vi "Move XYZ.vi"(0 "PID Gains In":T2={"X PID"={"proportional gain (Kc)"=0.03, "integral time (Ti, min)"=0.0, "derivative time (Td, min)"=0.0}, "Y PID"={"proportional gain (Kc)"=0.03, "integral time (Ti, min)"=0.0, "derivative time (Td, min)"=0.0}, "Z PID"={"proportional gain (Kc)"=0.035, "integral time (Ti, min)"=0.0, "derivative time (Td, min)"=0.0}} {"Z PID"."derivative time (Td, min)" format="%.3f"; "Z PID"."integral time (Ti, min)" format="%.3f"; "Z PID"."proportional gain (Kc)" format="%.3f"; "Y PID"."derivative time (Td, min)" format="%.3f"; "Y PID"."integral time (Ti, min)" format="%.3f"; "Y PID"."proportional gain (Kc)" format="%.3f"; "X PID"."derivative time (Td, min)" format="%.3f"; "X PID"."integral time (Ti, min)" format="%.3f"; "X PID"."proportional gain (Kc)" format="%.3f"}, 5 "Y Target":dbl, 6 "X Target":dbl, 10 "Max Time":dbl=90.0, 11 "Gyro Target":dbl=-180.0, 12 "Movement":dbl=3.0, 14 "X Output Range":cluster{"output high":dbl, "output low":dbl}={"output high"=0.8, "output low"=-0.8}, 15 "X Stop Threshold":dbl=5.0, 16 "Y Output Range":cluster{"output high":dbl, "output low":dbl}={"output high"=0.8, "output low"=-0.8}, 17 "Y Stop Threshold":dbl=5.0, 18 "Z Output Range":cluster{"output high":dbl, "output low":dbl}={"output high"=0.8, "output low"=-0.8}, 19 "Z  Stop Threshold":dbl=8.0) -> ()   [LabVIEW 2018]
uses:
  Robot Global Data.vi
  SubSystems/Drive Train/Drive Train Global.vi
  SubSystems/Hatch Panel Intake/Hatch Panel Intake Global.vi
  SubSystems/Lift/Lift Global.vi
  <vilib>/addons/control/pid/pid.llb/PID (DBL).vi
  <vilib>/addons/control/pid/NI_PID_pid.lvlib
panel:
  in  "Camera Tracking":T1={"proportional gain (Kc)"=0.06, "integral time (Ti, min)"=0.0, "derivative time (Td, min)"=0.0}
  in  "Minimum Time":u32=500
  in  "Settle Time":u32=2000
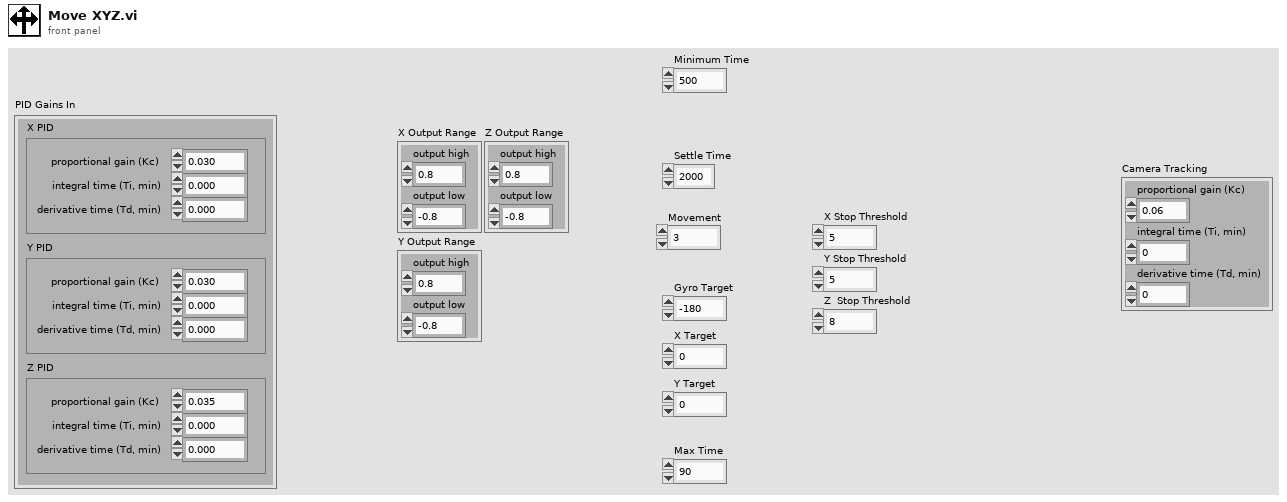
[diagram p1: front panel]
types:
  T1 = cluster{"proportional gain (Kc)":dbl, "integral time (Ti, min)":dbl, "derivative time (Td, min)":dbl}
  T2 = cluster{"X PID":cluster{"proportional gain (Kc)":dbl, "integral time (Ti, min)":dbl, "derivative time (Td, min)":dbl}, "Y PID":cluster{"proportional gain (Kc)":dbl, "integral time (Ti, min)":dbl, "derivative time (Td, min)":dbl}, "Z PID":cluster{"proportional gain (Kc)":dbl, "integral time (Ti, min)":dbl, "derivative time (Td, min)":dbl}}
  T3 = cluster{"Rollover":dbl, "Yaw":dbl, "Cont Yaw":dbl}
  T4 = cluster{"offsetAngle H":dbl, "offsetAngle V":dbl, "area":dbl, "skew":dbl, "validTarget":dbl, "latency":dbl}
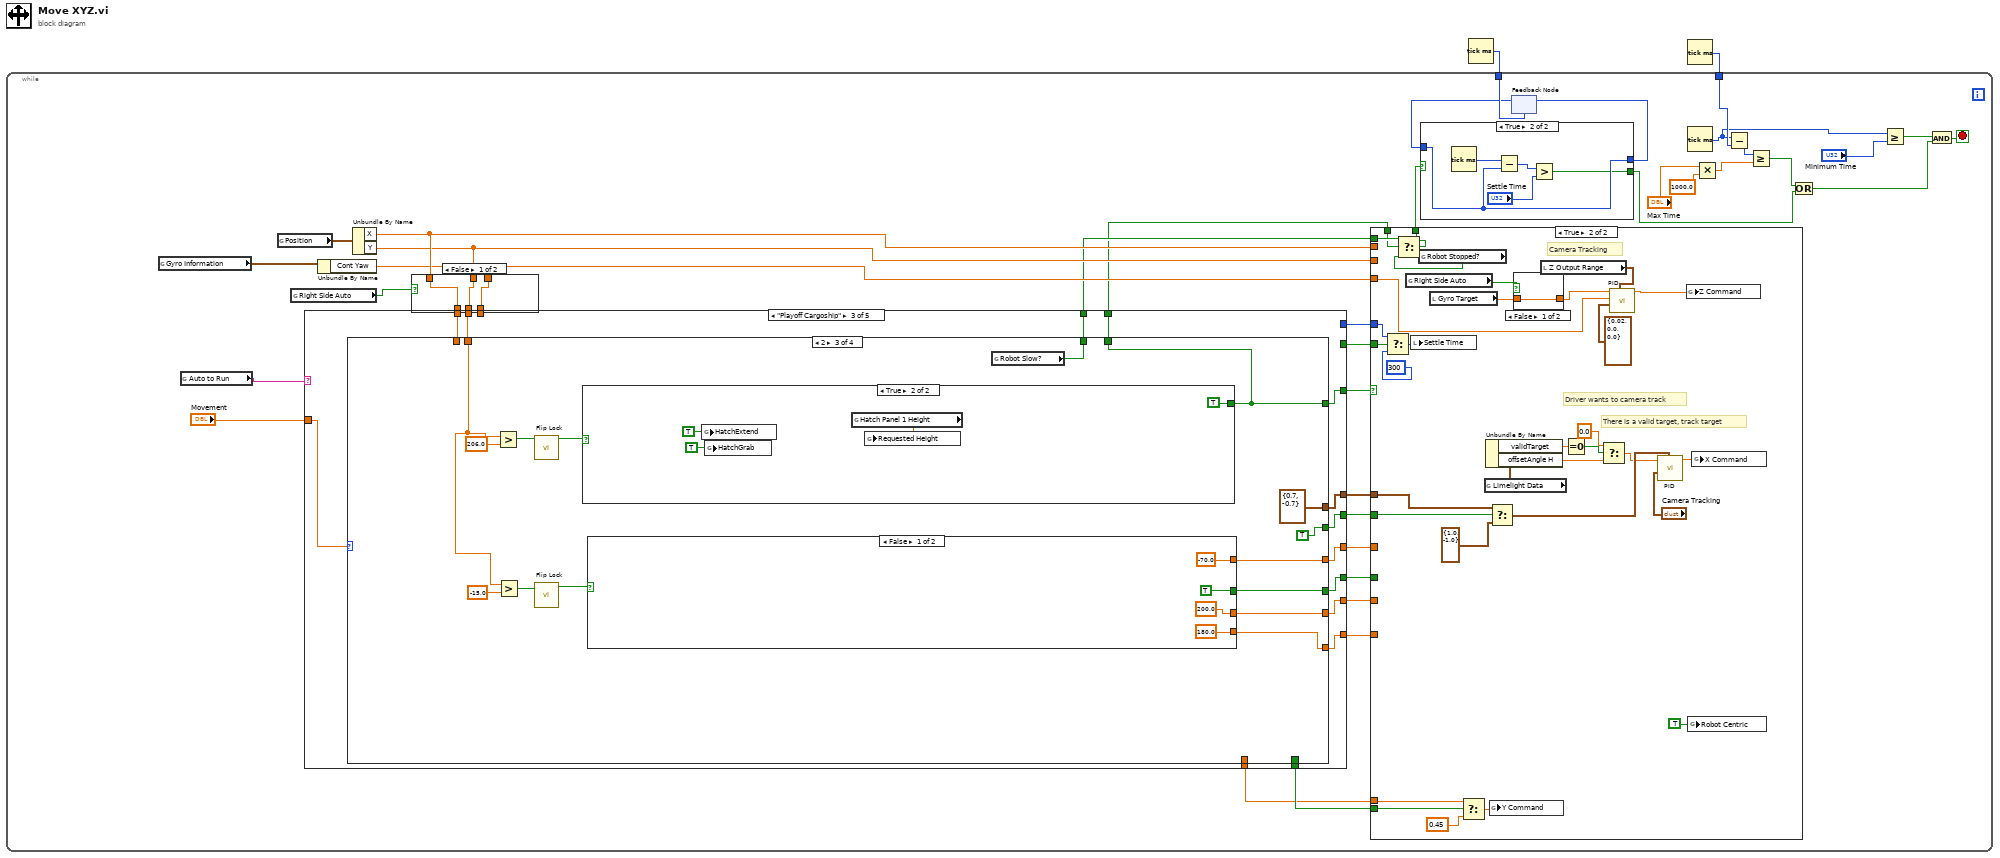
[diagram p0: block diagram]
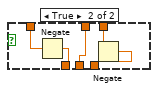
[diagram p2: hidden frame]
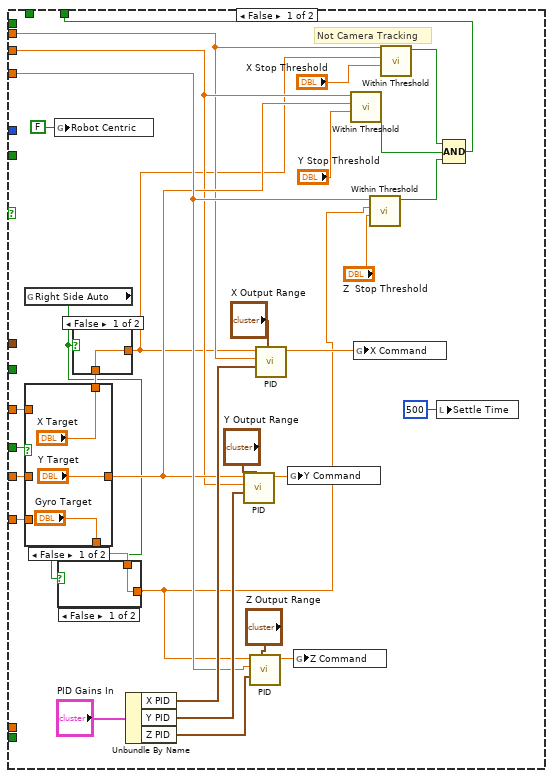
[diagram p3: hidden frame]
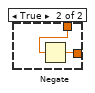
[diagram p4: hidden frame]
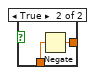
[diagram p5: hidden frame]
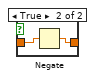
[diagram p7: hidden frame]
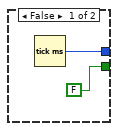
[diagram p8: hidden frame]
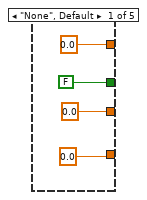
[diagram p9: hidden frame]
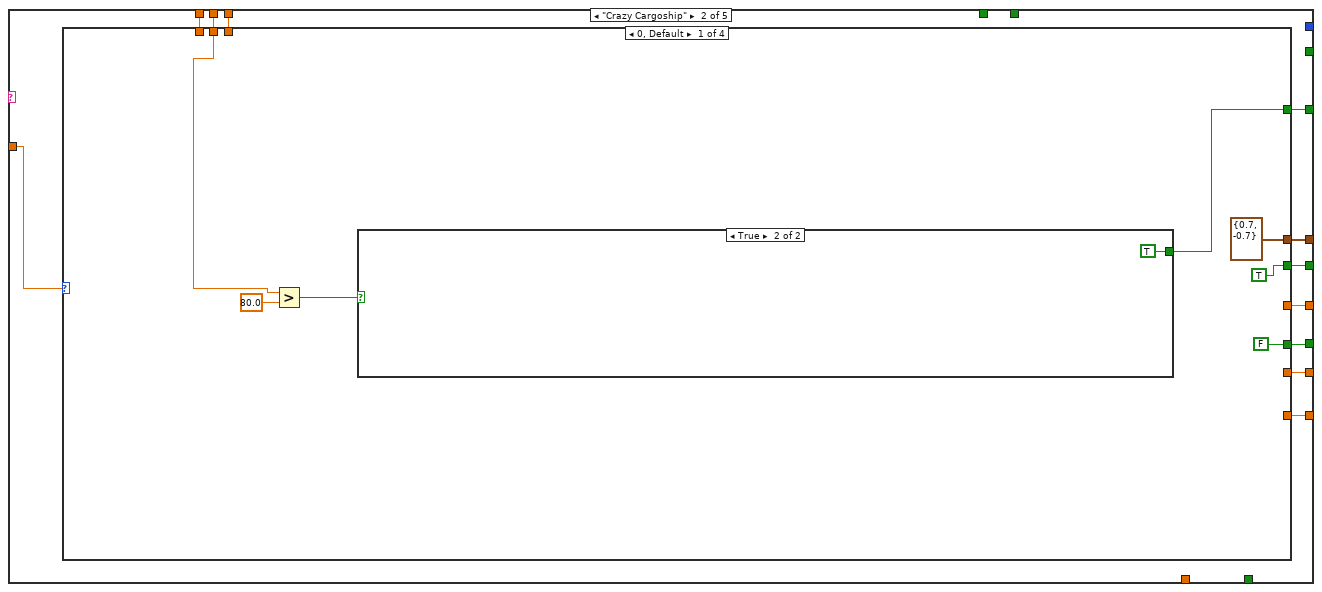
[diagram p10: hidden frame]
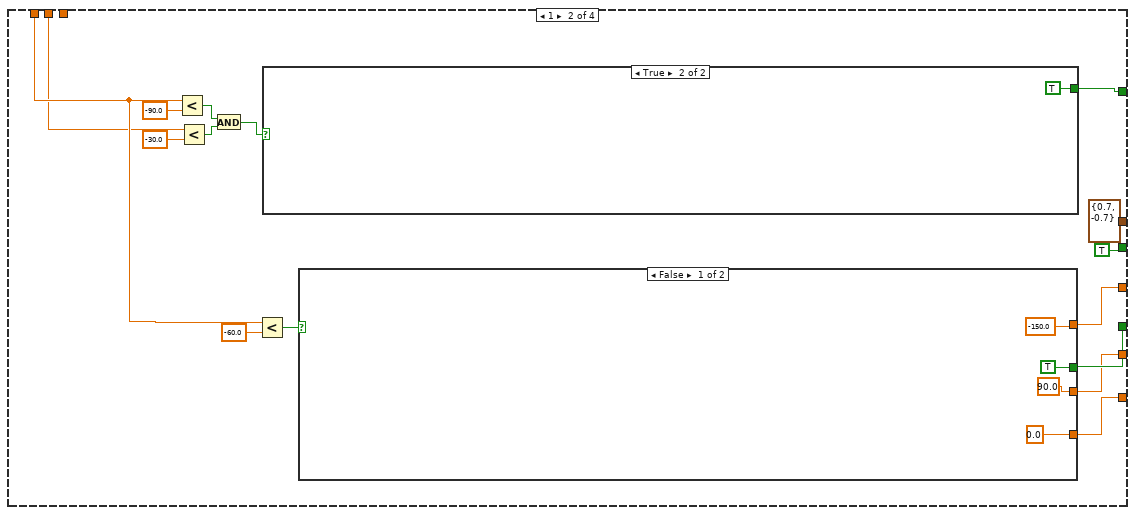
[diagram p12: hidden frame]
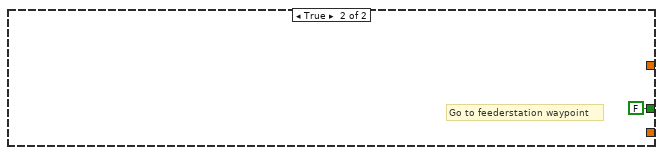
[diagram p13: hidden frame]
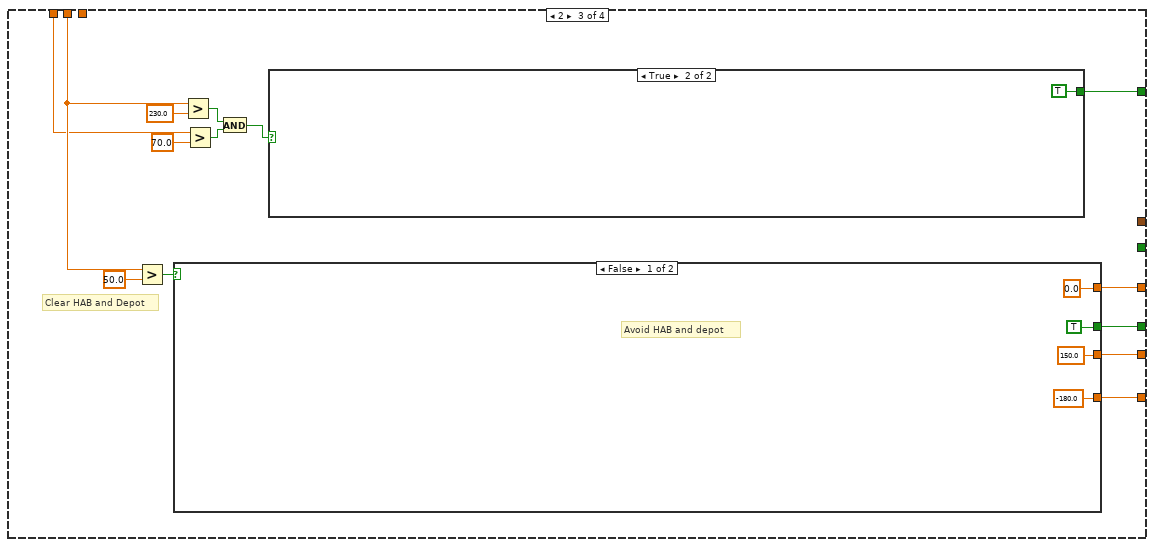
[diagram p15: hidden frame]
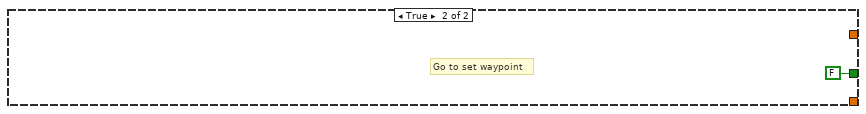
[diagram p17: hidden frame]
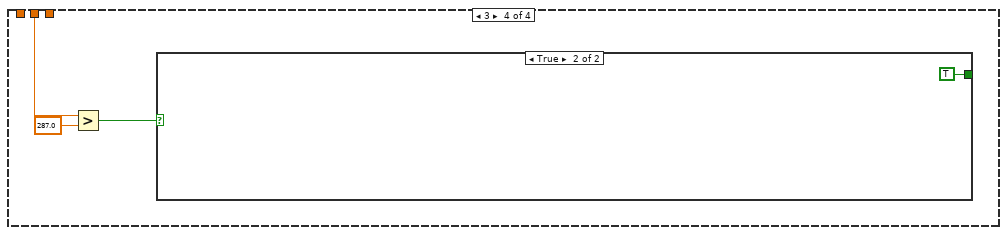
[diagram p18: hidden frame]
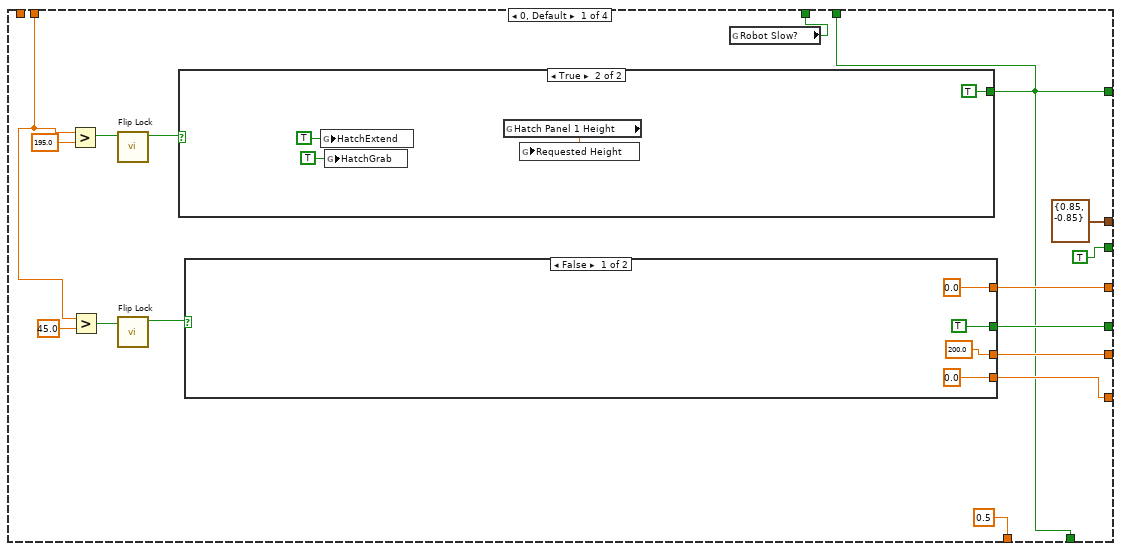
[diagram p20: hidden frame]
diagram:
  n1 = Tick Count (ms)() -> (millisecond timer value=w2:u32)
  n2 = Tick Count (ms)() -> (millisecond timer value=w1:u32)
  n3 = while {
    tunnel: w2 -> [w36]
    tunnel: w1 -> [w24]
    stop <- w23 stop-if-true
    n4 = global read "Drive Train Global.vi" "Gyro Information"() -> (w30:T3)
    n5 = global read "Robot Global Data.vi" "Auto to Run"() -> (w33:string)
    n6 = global read "Drive Train Global.vi" "Position"() -> (w32:cluster{"X":dbl, "Y":dbl})
    n7 = global read "Robot Global Data.vi" "Right Side Auto"() -> (w7:bool)
    n8 = Unbundle By Name(w30) -> ("Cont Yaw"=w9:dbl)
    n9 = Unbundle By Name(w32) -> ("X"=w12:dbl, "Y"=w10:dbl)
    n10 = case shown="False" w7 {
      tunnel: [w45 w50] -> w13
      tunnel: w12 -> [w45 w49]
      tunnel: [w44 w48] -> w11
      tunnel: w10 -> [w44 w48]
      tunnel: w9 -> [w43 w47]
      tunnel: [w43 w46] -> w8
      frame False {
      }
      frame True {
        n11 = Negate(x=w49) -> (-x=w50:dbl)
        n12 = Negate(x=w47) -> (-x=w46:dbl)
      }
    }
    n13 = case shown="\"Playoff Cargoship\"" w33 {
      tunnel: [0.0 w146 w213 w308 w403] -> w42
      tunnel: [0.0 w145 w211 w307 w402] -> w41
      tunnel: [0.0 w144 w210 w306 w401] -> w40
      tunnel: w11 -> [_ w150 w218 w311 w406]
      tunnel: [FALSE w149 w212 w309 w404] -> w39
      tunnel: w13 -> [_ w147 w219 w310 w405]
      tunnel: "Movement" -> [_ w151 w217 w312 w407]
      tunnel: w8 -> [_ w148 _ _ w399]
      tunnel: [_ w143 w215 w305 w400] -> w18
      tunnel: [_ w141 w216 w303 _] -> w17
      tunnel: [_ w142 w214 w304 _] -> w16
      tunnel: [_ _ _ w302 w398] -> w15
      tunnel: [_ _ _ w301 w397] -> w14
      tunnel: [_ _ w207 w300 _] -> w6
      tunnel: [_ _ w206 w299 _] -> w5
      tunnel: [_ _ w208 w298 _] -> w4
      tunnel: [_ _ w209 w297 _] -> w3
      frame "None", Default {
      }
      frame "Crazy Cargoship" {
        n14 = case shown="0, Default" w151 {
          tunnel: w150 -> [w154 w164 w183 w202]
          tunnel: [FALSE w175 w195 _] -> w149
          tunnel: w148 -> [_ _ _ _]
          tunnel: w147 -> [_ w165 w182 _]
          tunnel: [_ w174 w192 _] -> w146
          tunnel: [_ w173 w191 _] -> w145
          tunnel: [_ w172 w190 _] -> w144
          tunnel: [w156 w166 w184 _] -> w143
          tunnel: [TRUE ("Robot Centric") TRUE ("Robot Centric") _ _] -> w142
          tunnel: [cluster{"output high":dbl, "output low":dbl} {"output high"=0.7, "output low"=-0.7} ("output range") cluster{"output high":dbl, "output low":dbl} {"output high"=0.7, "output low"=-0.7} ("output range") _ _] -> w141
          frame 0, Default {
            n15 = Greater?(x=w154, y=80.0) -> (0:w155:bool)
            n16 = case shown="True" w155 {
              tunnel: [_ TRUE] -> w156
              frame False {
              }
              frame True {
              }
            }
          }
          frame 1 {
            n17 = Less?(x=w165, y=-90.0) -> (x < y?=w169:bool)
            n18 = Less?(x=w164, y=-30.0) -> (x < y?=w168:bool)
            n19 = And(x=w169, y=w168) -> (x .and. y?=w167:bool)
            n20 = Less?(x=w165, y=-60.0) -> (x < y?=w160:bool)
            n21 = case shown="True" w167 {
              tunnel: [_ TRUE] -> w166
              frame False {
              }
              frame True {
              }
            }
            n22 = case shown="False" w160 {
              tunnel: [TRUE FALSE] -> w175
              tunnel: [-150.0 _] -> w174
              tunnel: [90.0 _] -> w173
              tunnel: [0.0 _] -> w172
              frame False {
              }
              frame True {
                # "Go to feederstation waypoint"
              }
            }
          }
          frame 2 {
            # "Clear HAB and Depot"
            n23 = Greater?(x=w183, y=50.0) -> (0:w194:bool)
            n24 = case shown="False" w194 {
              tunnel: [TRUE FALSE] -> w195
              tunnel: [0.0 _] -> w192
              tunnel: [150.0 _] -> w191
              tunnel: [-180.0 _] -> w190
              frame False {
                # "Avoid HAB and depot"
              }
              frame True {
                # "Go to set waypoint"
              }
            }
            n25 = Greater?(x=w183, y=230.0) -> (0:w187:bool)
            n26 = Greater?(x=w182, y=70.0) -> (0:w186:bool)
            n27 = And(x=w187, y=w186) -> (x .and. y?=w185:bool)
            n28 = case shown="True" w185 {
              tunnel: [_ TRUE] -> w184
              frame False {
              }
              frame True {
              }
            }
          }
          frame 3 {
            n29 = Greater?(x=w202, y=287.0) -> (0:w203:bool)
            n30 = case shown="True" w203 {
              tunnel: [_ TRUE] -> _
              frame False {
              }
              frame True {
              }
            }
          }
        }
      }
      frame "Playoff Cargoship" {
        n31 = case shown="2" w217 {
          tunnel: w218 -> [w231 w246 w275 w289]
          tunnel: [w229 w249 w273 _] -> w212
          tunnel: w219 -> [_ _ _ _]
          tunnel: [w230 w250 w274 _] -> w213
          tunnel: [w228 w248 w272 _] -> w211
          tunnel: [w227 w247 w271 _] -> w210
          tunnel: [w220 w244 w266 w288] -> w215
          tunnel: [TRUE ("Robot Centric") _ TRUE ("Robot Centric") _] -> w214
          tunnel: [cluster{"output high":dbl, "output low":dbl} {"output high"=0.85, "output low"=-0.85} ("output range") _ cluster{"output high":dbl, "output low":dbl} {"output high"=0.7, "output low"=-0.7} ("output range") _] -> w216
          tunnel: [w220 w244 w266 _] -> w209
          tunnel: [w221 w245 w265 _] -> w208
          tunnel: [w220 _ _ _] -> w207
          tunnel: [0.5 ("Y Command") _ _ _] -> w206
          frame 0, Default {
            n32 = Greater?(x=w231, y=195.0) -> (0:w224:bool)
            n33 = Greater?(x=w231, y=45.0) -> (0:w226:bool)
            n34 = call "Flip Lock.vi"("Input"=w224) -> ("Output"=w223:bool)  [unwired: 10 in]
            n35 = call "Flip Lock.vi"("Input"=w226) -> ("Output"=w225:bool)  [unwired: 10 in]
            n36 = case shown="True" w223 {
              tunnel: [_ TRUE] -> w220
              frame False {
              }
              frame True {
                n37 = global write "Hatch Panel Intake Global.vi" "HatchExtend"(TRUE ("HatchExtend")) -> ()
                n38 = global write "Hatch Panel Intake Global.vi" "HatchGrab"(TRUE ("HatchGrab")) -> ()
                n39 = global read "Lift Global.vi" "Hatch Panel 1 Height"() -> (w242:dbl)
                n40 = global write "Lift Global.vi" "Requested Height"(w242) -> ()
              }
            }
            n41 = case shown="False" w225 {
              tunnel: [0.0 _] -> w230
              tunnel: [TRUE ("Robot Centric") _] -> w229
              tunnel: [200.0 _] -> w228
              tunnel: [0.0 _] -> w227
              frame False {
              }
              frame True {
              }
            }
            n42 = global read "Drive Train Global.vi" "Robot Slow?"() -> (w221:bool)
          }
          frame 1 {
            n43 = Less?(x=w246, y=15.0) -> (x < y?=w252:bool)
            n44 = Less?(x=w246, y=-5.0) -> (x < y?=w255:bool)
            n45 = call "Flip Lock.vi"("Input"=w252) -> ("Output"=w251:bool)  [unwired: 10 in]
            n46 = call "Flip Lock.vi"("Input"=w255) -> ("Output"=w254:bool)  [unwired: 10 in]
            n47 = case shown="True" w254 {
              tunnel: [_ TRUE] -> w244
              frame False {
              }
              frame True {
                n48 = global write "Hatch Panel Intake Global.vi" "HatchExtend"(TRUE ("HatchExtend")) -> ()
                n49 = global write "Hatch Panel Intake Global.vi" "HatchGrab"(FALSE ("HatchGrab")) -> ()
                n50 = global read "Lift Global.vi" "Hatch Panel 1 Height"() -> (w263:dbl)
                n51 = global write "Lift Global.vi" "Requested Height"(w263) -> ()
              }
            }
            n52 = case shown="False" w251 {
              tunnel: [-80.0 _] -> w250
              tunnel: [TRUE ("Robot Centric") _] -> w249
              tunnel: [-60.0 _] -> w248
              tunnel: [180.0 _] -> w247
              frame False {
              }
              frame True {
              }
            }
            n53 = global read "Drive Train Global.vi" "Robot Slow?"() -> (w245:bool)
          }
          frame 2 {
            n54 = Greater?(x=w275, y=206.0) -> (0:w268:bool)
            n55 = Greater?(x=w275, y=-15.0) -> (0:w270:bool)
            n56 = call "Flip Lock.vi"("Input"=w268) -> ("Output"=w267:bool)  [unwired: 10 in]
            n57 = call "Flip Lock.vi"("Input"=w270) -> ("Output"=w269:bool)  [unwired: 10 in]
            n58 = case shown="True" w267 {
              tunnel: [_ TRUE] -> w266
              frame False {
              }
              frame True {
                n59 = global write "Hatch Panel Intake Global.vi" "HatchExtend"(TRUE ("HatchExtend")) -> ()
                n60 = global write "Hatch Panel Intake Global.vi" "HatchGrab"(TRUE ("HatchGrab")) -> ()
                n61 = global read "Lift Global.vi" "Hatch Panel 1 Height"() -> (w286:dbl)
                n62 = global write "Lift Global.vi" "Requested Height"(w286) -> ()
              }
            }
            n63 = case shown="False" w269 {
              tunnel: [-70.0 _] -> w274
              tunnel: [TRUE ("Robot Centric") _] -> w273
              tunnel: [200.0 _] -> w272
              tunnel: [180.0 _] -> w271
              frame False {
              }
              frame True {
              }
            }
            n64 = global read "Drive Train Global.vi" "Robot Slow?"() -> (w265:bool)
          }
          frame 3 {
            n65 = Less?(x=w289, y=-30.0) -> (x < y?=w291:bool)
            n66 = call "Flip Lock.vi"("Input"=w291) -> ("Output"=w290:bool)  [unwired: 10 in]
            n67 = case shown="True" w290 {
              tunnel: [_ TRUE] -> w288
              frame False {
              }
              frame True {
                n68 = global write "Hatch Panel Intake Global.vi" "HatchExtend"(TRUE ("HatchExtend")) -> ()
                n69 = global write "Hatch Panel Intake Global.vi" "HatchGrab"(FALSE ("HatchGrab")) -> ()
                n70 = global read "Lift Global.vi" "Hatch Panel 1 Height"() -> (w295:dbl)
                n71 = global write "Lift Global.vi" "Requested Height"(w295) -> ()
              }
            }
          }
        }
      }
      frame "Fun Rocket Close" {
        n72 = case shown="0, Default" w312 {
          tunnel: w311 -> [w323 w343 w362 w385]
          tunnel: w310 -> [w324 w344 _ _]
          tunnel: [w328 _ w360 w380] -> w309
          tunnel: [w327 _ w361 w383] -> w308
          tunnel: [w326 _ w359 w382] -> w307
          tunnel: [w325 _ w358 w381] -> w306
          tunnel: [w316 w341 w357 w388] -> w305
          tunnel: [_ _ w366 _] -> w304
          tunnel: [_ _ w365 _] -> w303
          tunnel: [w316 w341 w357 _] -> w302
          tunnel: [u32 150 ("Settle Time") u32 150 ("Settle Time") u32 150 ("Settle Time") _] -> w301
          tunnel: [w316 TRUE _ _] -> w300
          tunnel: [0.6 ("Y Command") 0.4 ("Y Command") _ _] -> w299
          tunnel: [w314 w337 w354 w378] -> w298
          tunnel: [TRUE TRUE TRUE TRUE] -> w297
          frame 0, Default {
            # "Wait until robot gets off hab"
            n73 = Less?(x=w324, y=-35.0) -> (x < y?=w330:bool)
            n74 = Less?(x=w324, y=-70.0) -> (x < y?=w320:bool)
            n75 = Greater?(x=w323, y=50.0) -> (0:w319:bool)
            n76 = case shown="False" w330 {
              tunnel: [TRUE FALSE] -> w328
              tunnel: [-120.0 _] -> w327
              tunnel: [0.0 _] -> w326
              tunnel: [0.0 _] -> w325
              frame False {
                # "Go straight to the right off of the HAB"
              }
              frame True {
                # "Robot off of HAB, go to the rocket"
              }
            }
            n77 = And(x=w320, y=w319) -> (x .and. y?=w318:bool)
            n78 = case shown="True" w318 {
              tunnel: [_ TRUE] -> w316
              frame False {
              }
              frame True {
              }
            }
            n79 = global read "Drive Train Global.vi" "Robot Slow?"() -> (w314:bool)
          }
          frame 1 {
            n80 = Less?(x=w343, y=0.0) -> (x < y?=w347:bool)
            n81 = Less?(x=w344, y=10.0) -> (x < y?=w346:bool)
            n82 = And(x=w347, y=w346) -> (x .and. y?=w345:bool)
            n83 = case shown="True" w345 {
              tunnel: [_ TRUE] -> w341
              frame False {
              }
              frame True {
                n84 = global write "Hatch Panel Intake Global.vi" "HatchExtend"(TRUE ("HatchExtend")) -> ()
                n85 = global write "Hatch Panel Intake Global.vi" "HatchGrab"(FALSE ("HatchGrab")) -> ()
                n86 = global read "Lift Global.vi" "Hatch Panel 1 Height"() -> (w350:dbl)
                n87 = global write "Lift Global.vi" "Requested Height"(w350) -> ()
              }
            }
            n88 = global read "Drive Train Global.vi" "Robot Slow?"() -> (w337:bool)
          }
          frame 2 {
            # "back up then turn"
            n89 = Greater?(x=w362, y=150.0) -> (0:w367:bool)
            n90 = Greater?(x=w362, y=40.0) -> (0:w363:bool)
            n91 = case shown="True" w367 {
              tunnel: [_ TRUE] -> w357
              tunnel: [_ TRUE] -> w366
              tunnel: [_ cluster{"output high":dbl, "output low":dbl} {"output high"=0.6, "output low"=-0.6} ("output range")] -> w365
              frame False {
              }
              frame True {
                n92 = global read "Lift Global.vi" "Hatch Panel 1 Height"() -> (w374:dbl)
                n93 = global write "Lift Global.vi" "Requested Height"(w374) -> ()
              }
            }
            n94 = case shown="False" w363 {
              tunnel: [0.0 _] -> w361
              tunnel: [TRUE FALSE] -> w360
              tunnel: [200.0 _] -> w359
              tunnel: [-180.0 _] -> w358
              frame False {
              }
              frame True {
              }
            }
            n95 = global read "Drive Train Global.vi" "Robot Slow?"() -> (w354:bool)
          }
          frame 3 {
            n96 = Less?(x=w385, y=30.0) -> (x < y?=w387:bool)
            n97 = Less?(x=w385, y=140.0) -> (x < y?=w384:bool)
            n98 = case shown="True" w384 {
              tunnel: [0.0 _] -> w383
              tunnel: [100.0 _] -> w382
              tunnel: [-30.0 _] -> w381
              tunnel: [TRUE _] -> w380
              frame False {
              }
              frame True {
              }
            }
            n99 = case shown="True" w387 {
              tunnel: [_ TRUE] -> w388
              frame False {
              }
              frame True {
                n100 = global write "Hatch Panel Intake Global.vi" "HatchExtend"(TRUE ("HatchGrab")) -> ()
                n101 = global write "Hatch Panel Intake Global.vi" "HatchGrab"(FALSE ("HatchGrab")) -> ()
              }
            }
            n102 = global read "Drive Train Global.vi" "Robot Slow?"() -> (w378:bool)
          }
        }
      }
      frame "Fun Rocket Far" {
        n103 = case shown="1" w407 {
          tunnel: w406 -> [w413 w443 w478 w494]
          tunnel: w405 -> [w412 w450 _ _]
          tunnel: [w418 w448 w483 w489] -> w404
          tunnel: [w417 w449 w482 w492] -> w403
          tunnel: [w416 w447 w481 w491] -> w402
          tunnel: [w415 w446 w480 w490] -> w401
          tunnel: [w414 w452 _ w497] -> w400
          tunnel: w399 -> [_ _ _ _]
          tunnel: [w410 _ _ _] -> w398
          tunnel: [w411 _ _ _] -> w397
          frame 0, Default {
            # "Move to far rocket"
            # "Wait until robot gets off hab"
            n104 = Greater?(x=w413, y=210.0) -> (0:w408:bool)
            n105 = call "Flip Lock.vi"("Input"=w408) -> ("Output"=w409:bool)  [unwired: 10 in]
            n106 = case shown="True" w409 {
              tunnel: [TRUE w434] -> w418
              tunnel: [-10.0 w433] -> w417
              tunnel: [250.0 w432] -> w416
              tunnel: [0.0 w431] -> w415
              tunnel: [_ w430] -> w414
              tunnel: w412 -> [_ w428]
              tunnel: [_ w425] -> w411
              tunnel: [_ w424] -> w410
              frame False {
              }
              frame True {
                # "Wait for robot to be in good\nplace to camera track"
                n107 = Less?(x=w428, y=-80.0) -> (x < y?=w427:bool)
                n108 = call "Flip Lock.vi"("Input"=w427) -> ("Output"=w426:bool)  [unwired: 10 in]
                n109 = case shown="False" w426 {
                  tunnel: [TRUE FALSE] -> w434
                  tunnel: [-150.0 ("y") _] -> w433
                  tunnel: [230.0 ("y") _] -> w432
                  tunnel: [-130.0 ("y") _] -> w431
                  tunnel: [FALSE w440] -> w430
                  tunnel: [_ u32 500 ("Settle Time")] -> w425
                  tunnel: [_ w440] -> w424
                  frame False {
                  }
                  frame True {
                    w440 = TRUE
                  }
                }
              }
            }
          }
          frame 1 {
            n110 = Less?(x=w443, y=-30.0) -> (x < y?=w455:bool)
            n111 = Less?(x=w450, y=0.0) -> (x < y?=w454:bool)
            n112 = And(x=w455, y=w454) -> (x .and. y?=w453:bool)
            n113 = Greater?(x=w450, y=-60.0) -> (0:w444:bool)
            n114 = case shown="False" w453 {
              tunnel: [FALSE TRUE] -> w452
              frame False {
              }
              frame True {
              }
            }
            n115 = call "Flip Lock.vi"("Input"=w444) -> ("Output"=w445:bool)  [unwired: 10 in]
            n116 = case shown="True" w445 {
              tunnel: [0.0 ("y") w464] -> w449
              tunnel: [TRUE w465] -> w448
              tunnel: [230.0 ("y") w463] -> w447
              tunnel: [-150.0 ("y") w462] -> w446
              tunnel: w443 -> [_ w467]
              frame False {
              }
              frame True {
                n117 = Less?(x=w467, y=40.0) -> (x < y?=w468:bool)
                n118 = call "Flip Lock.vi"("Input"=w468) -> ("Output"=w469:bool)  [unwired: 10 in]
                n119 = case shown="True" w469 {
                  tunnel: [TRUE FALSE] -> w465
                  tunnel: [-70.0 ("y") _] -> w464
                  tunnel: [-40.0 ("y") _] -> w463
                  tunnel: [-180.0 ("y") _] -> w462
                  frame False {
                  }
                  frame True {
                  }
                }
              }
            }
          }
          frame 2 {
            n120 = Less?(x=w478, y=30.0) -> (x < y?=w479:bool)
            n121 = case shown="False" w479 {
              tunnel: [TRUE FALSE] -> w483
              tunnel: [-30.0 _] -> w482
              tunnel: [100.0 _] -> w481
              tunnel: [-180.0 _] -> w480
              frame False {
              }
              frame True {
              }
            }
          }
          frame 3 {
            n122 = Less?(x=w494, y=30.0) -> (x < y?=w496:bool)
            n123 = Less?(x=w494, y=140.0) -> (x < y?=w493:bool)
            n124 = case shown="False" w493 {
              tunnel: [0.0 _] -> w492
              tunnel: [100.0 _] -> w491
              tunnel: [-30.0 _] -> w490
              tunnel: [TRUE _] -> w489
              frame False {
              }
              frame True {
              }
            }
            n125 = case shown="True" w496 {
              tunnel: [_ TRUE] -> w497
              frame False {
              }
              frame True {
              }
            }
          }
        }
      }
    }
    n126 = case shown="True" w18 {
      tunnel: w42 -> [w75 _]
      tunnel: w41 -> [w74 _]
      tunnel: w40 -> [w73 _]
      tunnel: w39 -> [w72 _]
      tunnel: [w58 w98] -> w29
      tunnel: w9 -> [w67 w122]
      tunnel: w10 -> [w63 _]
      tunnel: w12 -> [w60 _]
      tunnel: w17 -> [_ w118]
      tunnel: w16 -> [_ w117]
      tunnel: w15 -> [_ w114]
      tunnel: w14 -> [_ w113]
      tunnel: w6 -> [_ w101]
      tunnel: w5 -> [_ w100]
      tunnel: w4 -> [_ w97]
      tunnel: w3 -> [_ w96]
      frame False {
        # "Not Camera Tracking"
        n127 = global read "Robot Global Data.vi" "Right Side Auto"() -> (w51:bool)
        n128 = case shown="False" w72 {
          tunnel: ["X Target" w94] -> w55
          tunnel: ["Y Target" w93] -> w64
          tunnel: ["Gyro Target" w92] -> w53
          tunnel: w75 -> [_ w94]
          tunnel: w74 -> [_ w93]
          tunnel: w73 -> [_ w92]
          frame False {
          }
          frame True {
          }
        }
        n129 = global write "Drive Train Global.vi" "Robot Centric"(FALSE ("Robot Centric")) -> ()
        n130 = case shown="False" w51 {
          tunnel: w53 -> [w83 w84]
          tunnel: [w83 w85] -> w52
          frame False {
          }
          frame True {
            n131 = Negate(x=w84) -> (-x=w85:dbl)
          }
        }
        n132 = case shown="False" w51 {
          tunnel: w55 -> [w86 w87]
          tunnel: [w86 w88] -> w54
          frame False {
          }
          frame True {
            n133 = Negate(x=w87) -> (-x=w88:dbl)
          }
        }
        n134 = Unbundle By Name("PID Gains In") -> ("X PID"=w80:T1, "Y PID"=w79:T1, "Z PID"=w78:T1)
        n135 = call-poly <vilib>:"PID.vi"("output range"="Y Output Range", "PID gains"=w79, "process variable"=w63, "setpoint"=w64) -> ("output"=w69:dbl)  [unwired: 6 in, 1 out]
        n136 = call-poly <vilib>:"PID.vi"("output range"="Z Output Range", "PID gains"=w78, "process variable"=w67, "setpoint"=w52) -> ("output"=w70:dbl)  [unwired: 6 in, 1 out]
        n137 = call-poly <vilib>:"PID.vi"("output range"="X Output Range", "PID gains"=w80, "process variable"=w60, "setpoint"=w54) -> ("output"=w71:dbl)  [unwired: 6 in, 1 out]
        n138 = global write "Drive Train Global.vi" "Y Command"(w69) -> ()
        n139 = global write "Drive Train Global.vi" "Z Command"(w70) -> ()
        n140 = call "Within Threshold.vi"("Threshold"="Y Stop Threshold", "Center"=w64, "Value"=w63) -> ("Within Threshold?"=w65:bool)  [unwired: 8 in]
        n141 = global write "Drive Train Global.vi" "X Command"(w71) -> ()
        n142 = call "Within Threshold.vi"("Threshold"="Z  Stop Threshold", "Center"=w52, "Value"=w67) -> ("Within Threshold?"=w68:bool)  [unwired: 8 in]
        n143 = call "Within Threshold.vi"("Threshold"="X Stop Threshold", "Center"=w54, "Value"=w60) -> ("Within Threshold?"=w61:bool)  [unwired: 8 in]
        n144 = local write "Settle Time"(u32 500 ("Settle Time")) -> ()
        n145 = Compound Arithmetic op=AND(w61, w65, w68) -> (w58:bool)
      }
      frame True {
        # "There is a valid target, track target"
        # "Driver wants to camera track"
        # "Camera Tracking"
        n146 = Select(t=w113, s=w114, f=u32 300 ("Settle Time")) -> (s? t:f=w116:u32)
        n147 = global read "Robot Global Data.vi" "Right Side Auto"() -> (w105:bool)
        n148 = local write "Settle Time"(w116) -> ()
        n149 = global read "Drive Train Global.vi" "Robot Stopped?"() -> (w99:bool)
        n150 = Select(t=w97, s=w96, f=w99) -> (s? t:f=w98:bool)
        n151 = local read "Gyro Target"() -> (w107:dbl)
        n152 = Select(t=w100, s=w101, f=0.45 ("Y Command")) -> (s? t:f=w103:dbl)
        n153 = global read "Robot Global Data.vi" "Limelight Data"() -> (w125:T4)
        n154 = Unbundle By Name(w125) -> ("validTarget"=w112:dbl, "offsetAngle H"=w111:dbl)
        n155 = global write "Drive Train Global.vi" "Y Command"(w103) -> ()
        n156 = Select(t=w118, s=w117, f=cluster{"output high":dbl, "output low":dbl} {"output high"=1.0, "output low"=-1.0} ("output range")) -> (s? t:f=w119:cluster{"output high":dbl, "output low":dbl})
        n157 = case shown="False" w105 {
          tunnel: w107 -> [w127 w128]
          tunnel: [w127 w129] -> w106
          frame False {
          }
          frame True {
            n158 = Negate(x=w128) -> (-x=w129:dbl)
          }
        }
        n159 = local read "Z Output Range"() -> (w123:cluster{"output high":dbl, "output low":dbl})
        n160 = Equal To 0?(x=w112) -> (x = 0?=w109:bool)
        n161 = Select(t=0.0, s=w109, f=w111) -> (s? t:f=w110:dbl)
        n162 = call-poly <vilib>:"PID.vi"("output range"=w123, "PID gains"=T1 {"proportional gain (Kc)"=0.02, "integral time (Ti, min)"=0.0, "derivative time (Td, min)"=0.0}, "process variable"=w122, "setpoint"=w106) -> ("output"=w104:dbl)  [unwired: 6 in, 1 out]
        n163 = call-poly <vilib>:"PID.vi"("output range"=w119, "PID gains"="Camera Tracking", "setpoint"=w110) -> ("output"=w126:dbl)  [unwired: 7 in, 1 out]
        n164 = global write "Drive Train Global.vi" "Z Command"(w104) -> ()
        n165 = global write "Drive Train Global.vi" "Robot Centric"(TRUE ("Robot Centric")) -> ()
        n166 = global write "Drive Train Global.vi" "X Command"(w126) -> ()
      }
    }
    n167 = feedback #1(w36) -> (w35:u32)
    n168 = case shown="True" w29 {
      tunnel: [w131 w134] -> w37
      tunnel: w35 -> [_ w134]
      tunnel: [FALSE w133] -> w34
      frame False {
        n169 = Tick Count (ms)() -> (millisecond timer value=w131:u32)
      }
      frame True {
        n170 = Tick Count (ms)() -> (millisecond timer value=w136:u32)
        n171 = Subtract(x=w136, y=w134) -> (x-y=w135:u32)
        n172 = Greater?(x=w135, y="Settle Time") -> (0:w133:bool)
      }
    }
    n173 = feedback-in #1(w37) -> ()
    n174 = Tick Count (ms)() -> (millisecond timer value=w22:u32)
    n175 = Multiply(x="Max Time", y=1000.0) -> (x*y=w27:dbl)
    n176 = Subtract(x=w22, y=w24) -> (x-y=w28:u32)
    n177 = Greater Or Equal?(x=w28, y=w27) -> (x >= y?=w38:bool)
    n178 = Or(x=w38, y=w34) -> (x .or. y?=w19:bool)
    n179 = Greater Or Equal?(x=w22, y="Minimum Time") -> (x >= y?=w20:bool)
    n180 = And(x=w20, y=w19) -> (x .and. y?=w23:bool)
  }
